vi "Configure Gate Time.vi"(8 "error in (no error)":errorcluster, 10 "Select Gate Time (0.01)":i8(ring) items=["0.01", "0.1", "1", "10"], 11 "VISA resource name":refnum<visa-resource-name>) -> (0 "error out":errorcluster, 3 "VISA resource name out":refnum<visa-resource-name>)   [LabVIEW 2019, in "BK Precision 1823A.lvlib"]
doc: "This VI controls the gate time of the counter. Gate time is not applicable in \"Total\" function. <b>Select Gate Time</b> allows controllability of the gate time. Input integer value of 0 for 0.01 seconds, 1 for 0.1 seconds, 2 for 1 second, and 3 for 10 seconds gate time."
uses:
  BK Precision 1823A.lvlib
panel:
  # "(c) 2009 B&K PRECISION CORPORATION.  ALL RIGHTS RESERVED."
  # "seconds"
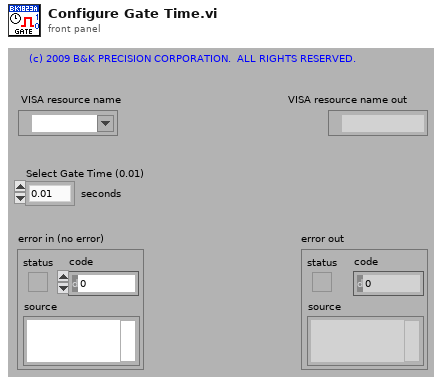
[diagram p1: front panel]
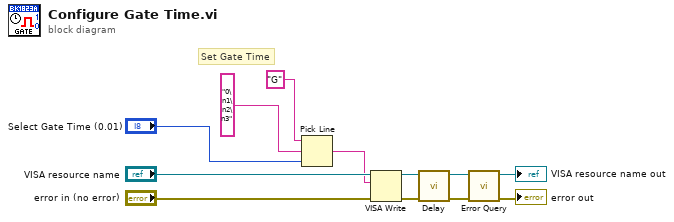
[diagram p0: block diagram]
diagram:
  # "Set Gate Time"
  n1 = Pick Line(string ("")="G", multi-line string="0\n1\n2\n3", line index="Select Gate Time (0.01)") -> (output string=w5:string)
  n2 = VISA Write(VISA resource name="VISA resource name", write buffer=w5, error in (no error)="error in (no error)") -> (VISA resource name out=w3:refnum<visa-resource-name>, error out=w4:errorcluster)  [unwired: 1 out]
  n3 = call "Delay.vi"("error in (no error)"=w4, "VISA resource name"=w3) -> ("error out"=w1:errorcluster, "VISA resource name out"=w2:refnum<visa-resource-name>)  [unwired: 8 in]
  n4 = call "Error Query.vi"("error in (no error)"=w1, "VISA resource name"=w2) -> ("error out"=→"error out":errorcluster, "VISA resource name out"=→"VISA resource name out":refnum<visa-resource-name>)  [unwired: 8 in]
